vi "Vision - Scaling Split.vi"(10 "Rails":dbl=2.0, 11 "ThumbNail Dims in":T1) -> (3 "ThumbNail Dims out":T1)   [LabVIEW 2024]
uses:
  Controls/ThumbNail Dimensions.ctl
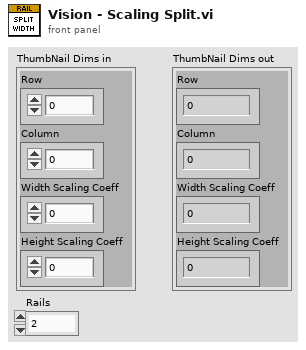
[diagram p1: front panel]
types:
  T1 = typedef "ThumbNail Dimensions.ctl" = cluster{"Row":i32, "Column":i32, "Width Scaling Coeff":dbl, "Height Scaling Coeff":dbl}
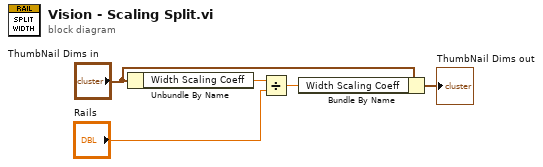
[diagram p0: block diagram]
diagram:
  n1 = Unbundle By Name("ThumbNail Dims in") -> ("Width Scaling Coeff"=w4:dbl)
  n2 = Divide(x=w4, y="Rails") -> (x/y=w2:dbl)
  n3 = Bundle By Name(cluster="ThumbNail Dims in", "Width Scaling Coeff"=w2) -> (→"ThumbNail Dims out":T1)
